vi "JTAG ADCScope.vi"() -> ()   [LabVIEW 2009]
panel:
  in  "stop 2":bool
  in  "Sample-Input Polarity":enum16{"Non-Inverted", "Inverted"}(ring)
  in  "Sample-Input Source Select":T1(ring)
  in  "ADC12 Clock Divider":T2(ring)
  in  "ADC12 Clock Source":enum16{"ADC12OSC", "ACLK", "MCLK", "SMCLK"}(ring)=enum."MCLK"
  in  "Update Delay (mS)":u32=100
  in  "Sample-Hold Trigger Source":enum16{"Sample-Input Signal", "Sampling Timer"}(ring)=enum."Sampling Timer"
  in  "MEM8-MEM15":T3(ring)
  in  "MEM0-MEM7":T3(ring)
  in  "Reference Generator":T4(ring)
  in  "Tab Control":enum32{"Single Channel", "Quad Channel"}(tab)
  out "ARG 7S":u16 format="%04x"
  out "Waveform Chart - Single Channel":u16(graph)
  in  "Select Voltage References (MEM0 Single)":T5(ring)
  in  "Input Channel Select (MEM0 Single)":T6(ring)
  in  "Select Voltage References (MEM3)":T5(ring)
  in  "Input Channel Select (MEM3)":T6(ring)
  in  "Select Voltage References (MEM2)":T5(ring)
  in  "Input Channel Select (MEM2)":T6(ring)
  in  "Select Voltage References (MEM1)":T5(ring)
  in  "Input Channel Select (MEM1)":T6(ring)
  out "Waveform Chart - 4 Channel":cluster{u16, u16, u16, u16}(graph)
  in  "Select Voltage References (MEM0)":T5(ring)
  in  "Input Channel Select (MEM0)":T6(ring)
  out "ARG 7M":u16 format="%04x"
  out "ARG 6M":u16 format="%04x"
  out "ARG 5M":u16 format="%04x"
  out "ARG 4M":u16 format="%04x"
  in  "stop":bool
  # "Sample and Hold Duration (ADC12 Clocks)"
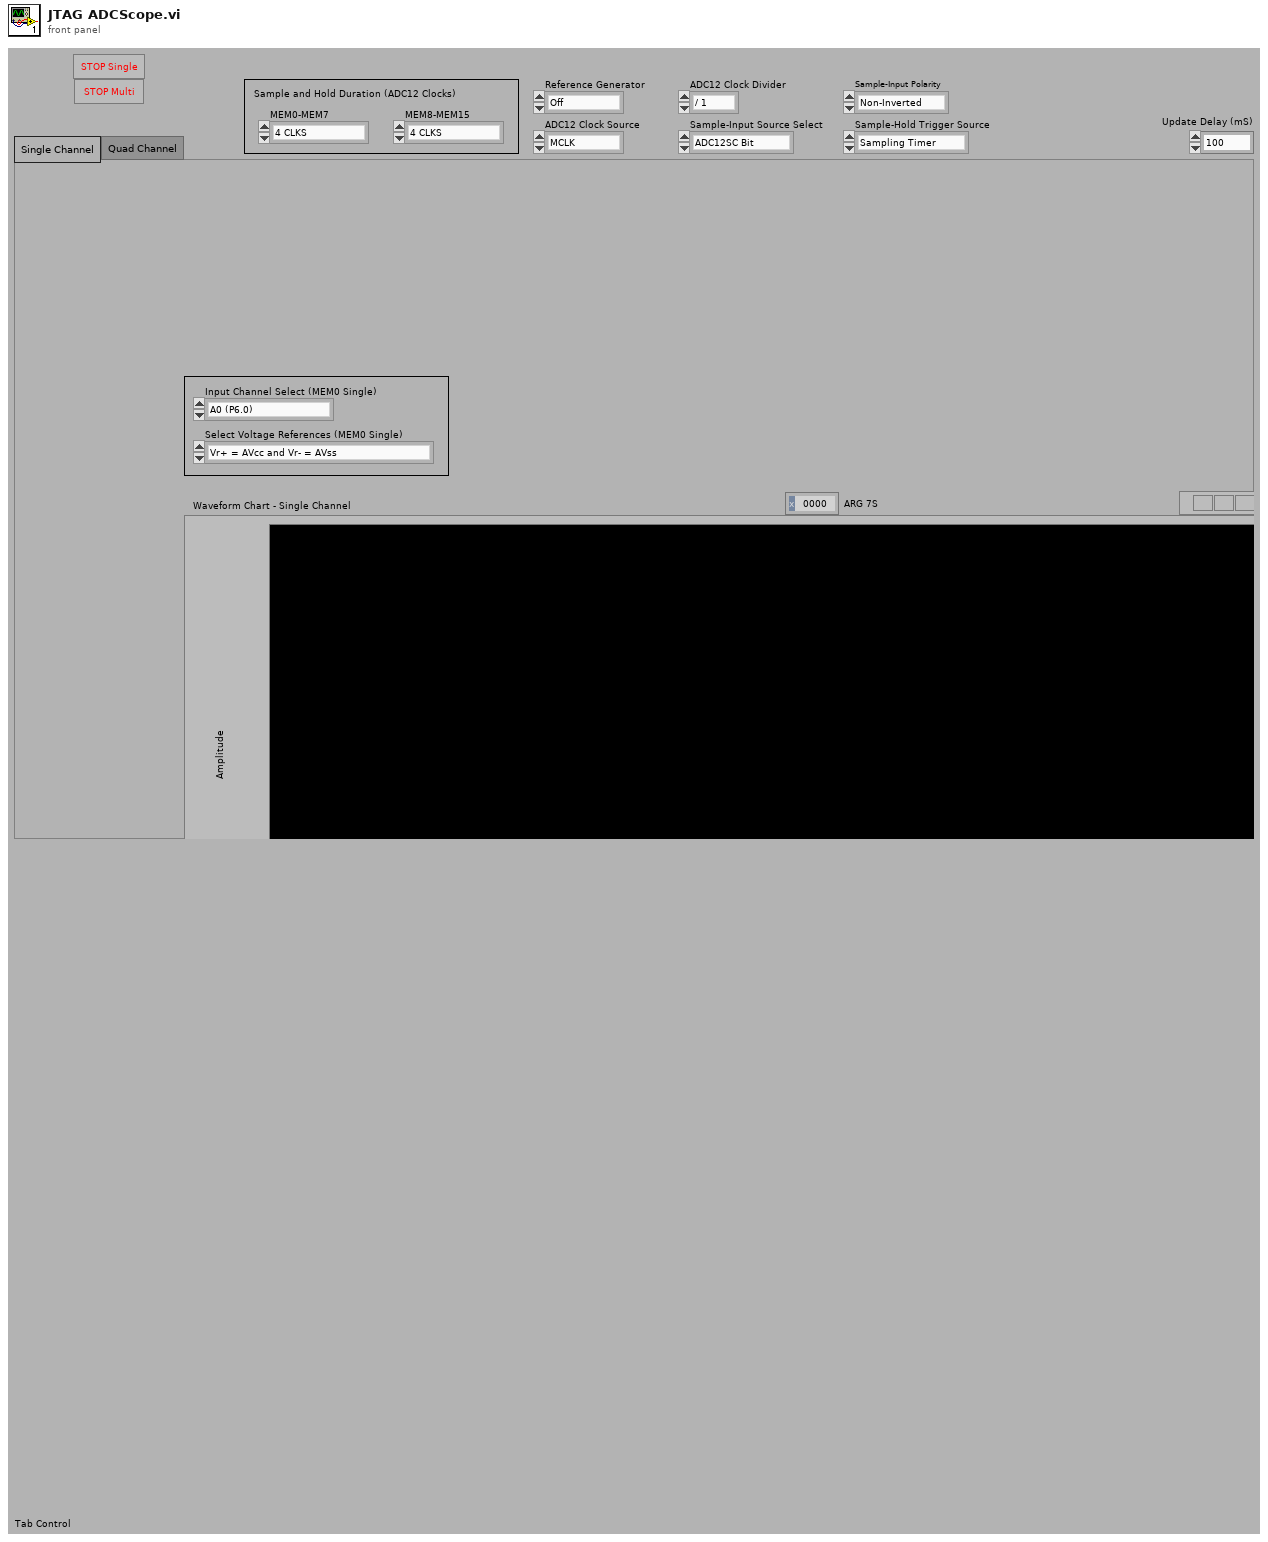
[diagram p1: front panel]
types:
  T1 = enum16{"ADC12SC Bit", "Timer_A OUT1", "Timer_B OUT0", "Timer_B OUT1"}
  T2 = enum16{"/ 1", "/ 2", "/ 3", "/ 4", "/ 5", "/ 6", "/ 7", "/ 8"}
  T3 = enum16{"4 CLKS", "8 CLKS", "16 CLKS", "32 CLKS", "64 CLKS", "96 CLKS", "128 CLKS", "192 CLKS", "256 CLKS", "384 CLKS", "512 CLKS", "768 CLKS", "1024 CLKS", "1024 CLKS (13)", "1024 CLKS (14)", "1024 CLKS (15)"}
  T4 = enum16{"Off", "ON - 1.5 V", "Off (2)", "ON - 2.5 V"}
  T5 = enum16{"Vr+ = AVcc and Vr- = AVss", "Vr+ = Vref+ and Vr-  = AVss", "Vr+ = Ve ref+ and Vr- = AVss", "Vr+ = Ve ref+ and Vr- = AVss (3)", "Vr+ = AVcc and Vr- = Vref- / Ve ref-", "Vr+ = Vref+ and Vr- = Vref- / Ve ref-", "Vr+ = Ve ref+ and Vr- = Vref- / Ve ref-", "Vr+ = Ve ref+ and Vr- = Vref- / Ve ref- (7)"}
  T6 = enum16{"A0 (P6.0)", "A1 (P6.1)", "A2 (P6.2)", "A3 (P6.3)", "A4 (P6.4)", "A5 (P6.5)", "A6 (P6.6)", "A7 (P6.7)", "Ve ref+", "V ref- / Ve ref-", "Temperature Diode", "(AVcc - AVss) / 2", "GND", "GND (13)", "GND (14)", "GND (15)"}
  T7 = enum8{"PORT_OUT", "PORT_SEL", "PORT_RES_EN", "READ_PORT", "PORT_DIR", "SET_LCM", "PLUTO_WRITE_SINGLE", "PLUTO_READ_SINGLE", "PLUTO_WRITE_MASK", "STIM_POWER_UP", "STIM_POWER_DN", "SATURN_WRITE_SINGLE", "SATURN_READ_SINGLE", "SATURN_WRITE_BLOCK", "SATURN_READ_BLOCK", "SATURN_WRITE_MASK", "MICS_POWER_UP", "MICS_POWER_DN", "MICS_WRITE_SINGLE", "MICS_READ_SINGLE", "MICS_WRITE_BLOCK", "MICS_READ_BLOCK", "MICS_WRITE_MASK", "MEM_POWER_UP", "MEM_POWER_DN", "MEM_WRITE_SINGLE", "MEM_READ_SINGLE", "MEM_WRITE_BLOCK", "MEM_READ_BLOCK", "MEM_WRITE_MASK", "MEM_WRITE_SR", "MEM_READ_SR", "MEM_OPCODE", "INIT_VARIABLES", "DCO -> 1 MHz", "DCO -> 8 MHz", "START_STIM_CLK", "STOP_STIM_CLK", "PULSE_STIM_CLK", "PULSE_STIM_SCK", "SINGLE_ADC12", "SINGLE_ADC12_REPEAT", "MULTI_ADC12", "MULTI_ADC12_REPEAT", "Disable_ADC12", "READ_IO_VARIABLES"}
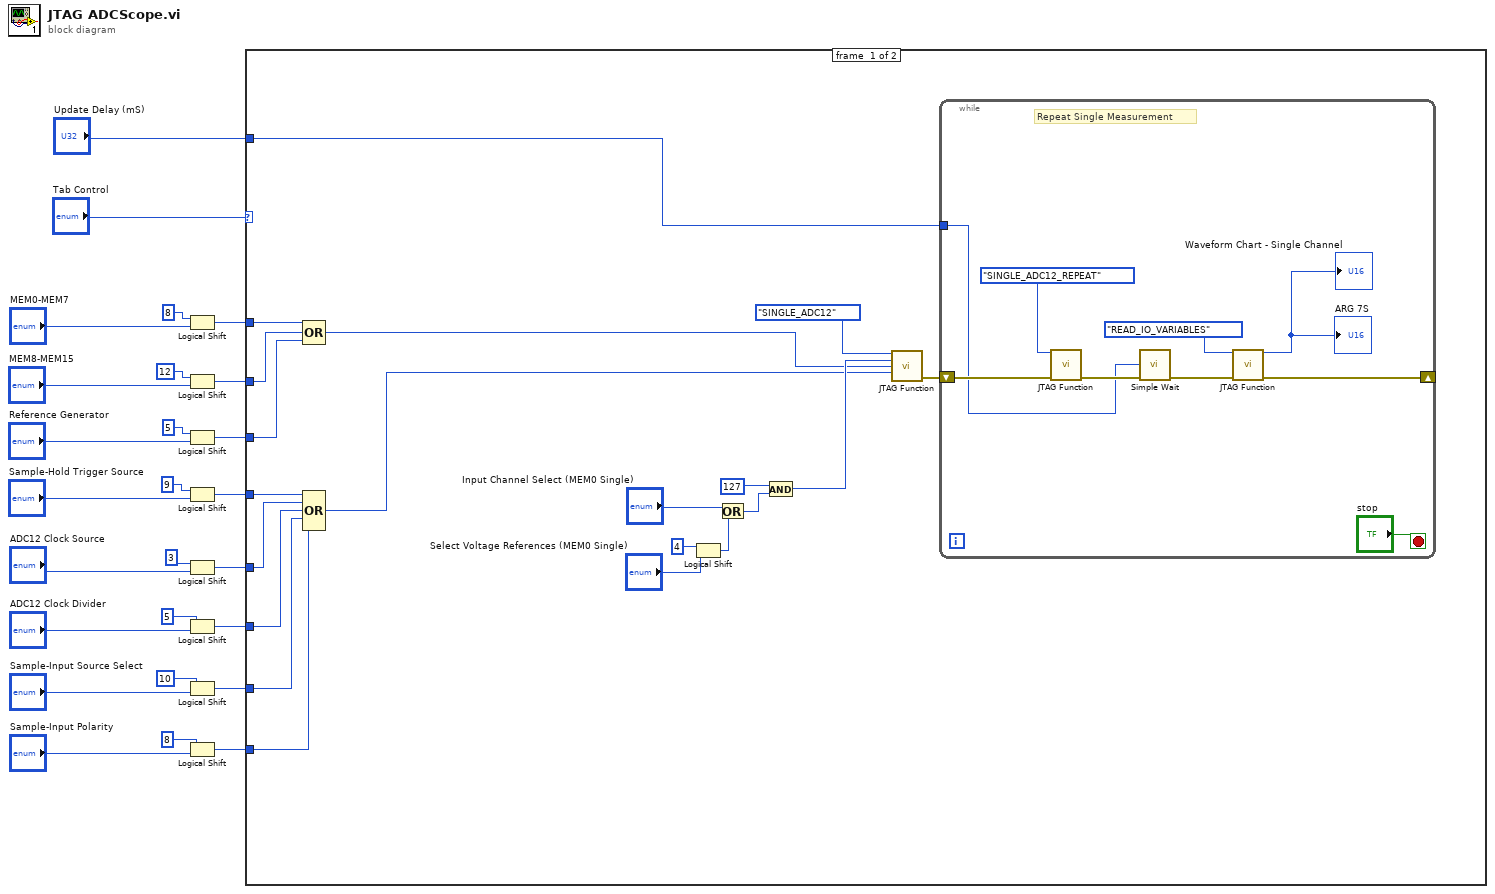
[diagram p0: block diagram]
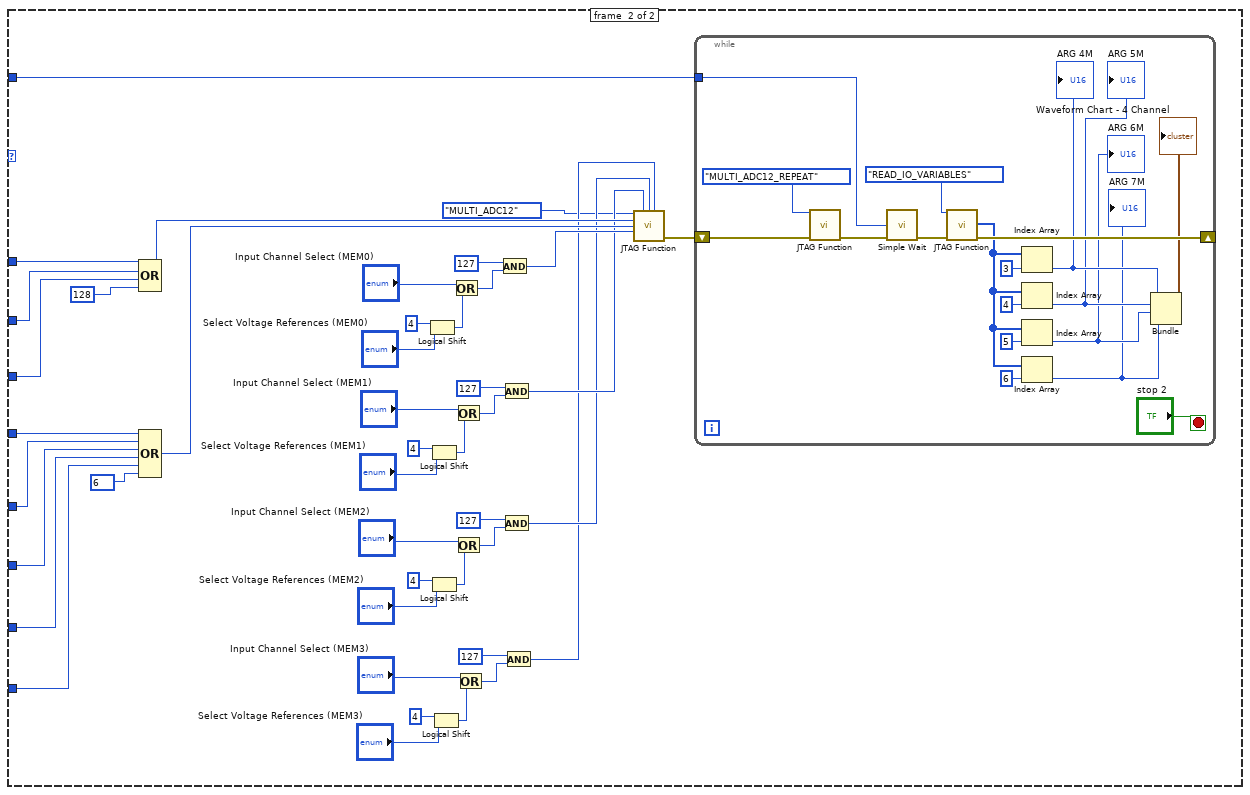
[diagram p2: hidden frame]
diagram:
  n1 = Logical Shift(y=i16 8, x="MEM0-MEM7") -> (x << y=w16:u32)
  n2 = Logical Shift(y=i16 12, x="MEM8-MEM15") -> (x << y=w15:u32)
  n3 = Logical Shift(y=i16 5, x="Reference Generator") -> (x << y=w14:u32)
  n4 = Logical Shift(y=i16 9, x="Sample-Hold Trigger Source") -> (x << y=w5:u32)
  n5 = Logical Shift(y=i16 3, x="ADC12 Clock Source") -> (x << y=w1:u32)
  n6 = Logical Shift(y=i16 5, x="ADC12 Clock Divider") -> (x << y=w2:u32)
  n7 = Logical Shift(y=i16 10, x="Sample-Input Source Select") -> (x << y=w3:u32)
  n8 = Logical Shift(y=i16 8, x="Sample-Input Polarity") -> (x << y=w4:u32)
  n9 = case shown="\"Single Channel\", Default" "Tab Control" {
    tunnel: "Update Delay (mS)" -> [w46 w98]
    tunnel: w16 -> [w39 w97]
    tunnel: w15 -> [w38 w96]
    tunnel: w14 -> [w37 w95]
    tunnel: w5 -> [w36 w94]
    tunnel: w4 -> [w35 w90]
    tunnel: w3 -> [w34 w91]
    tunnel: w2 -> [w33 w92]
    tunnel: w1 -> [w32 w93]
    frame #0 {
      n10 = Compound Arithmetic op=OR(w39, w38, w37) -> (w30:u32)
      n11 = Compound Arithmetic op=OR(w36, w32, w33, w34, w35) -> (w29:u32)
      n12 = Logical Shift(y=i16 4, x="Select Voltage References (MEM0 Single)") -> (x << y=w40:u32)
      n13 = Or(x="Input Channel Select (MEM0 Single)", y=w40) -> (x .or. y?=w44:u32)
      n14 = And(x=u8 127, y=w44) -> (x .and. y?=w31:u32)
      n15 = call "JTAG Function.vi"("Enum"=T7."SINGLE_ADC12", "ARG 1"=w31, "ARG 2"=w30, "ARG 3"=w29) -> ("error out"=w28:errorcluster)  [unwired: 9 in, 2 out]
      n16 = while {
        tunnel: w46 -> [w49]
        shift-right: [w54] -> _
        shift-left: w28 -> [w53]
        stop <- "stop" stop-if-true
        # "Repeat Single Measurement"
        n17 = call "JTAG Function.vi"("Enum"=T7."SINGLE_ADC12_REPEAT", "error in (no error)"=w53) -> ("error out"=w51:errorcluster)  [unwired: 11 in, 2 out]
        n18 = call "Simple Wait.vi"("mS"=w49, "error in"=w51) -> ("error out"=w50:errorcluster)  [unwired: 12 in, 1 out]
        n19 = call "JTAG Function.vi"("Enum"=T7."READ_IO_VARIABLES", "error in (no error)"=w50) -> ("ARG 7"=→"ARG 7S" →"Waveform Chart - Single Channel":u16, "error out"=w54:errorcluster)  [unwired: 11 in, 1 out]
      }
    }
    frame #1 {
      n20 = Compound Arithmetic op=OR(w97, w96, w95, u16 128) -> (w88:u32)
      n21 = Compound Arithmetic op=OR(w94, w93, w92, w91, w90, u16 6) -> (w87:u32)
      n22 = Logical Shift(y=i16 4, x="Select Voltage References (MEM0)") -> (x << y=w83:u32)
      n23 = Logical Shift(y=i16 4, x="Select Voltage References (MEM1)") -> (x << y=w79:u32)
      n24 = Logical Shift(y=i16 4, x="Select Voltage References (MEM2)") -> (x << y=w75:u32)
      n25 = Logical Shift(y=i16 4, x="Select Voltage References (MEM3)") -> (x << y=w71:u32)
      n26 = Or(x="Input Channel Select (MEM0)", y=w83) -> (x .or. y?=w85:u32)
      n27 = Or(x="Input Channel Select (MEM1)", y=w79) -> (x .or. y?=w81:u32)
      n28 = Or(x="Input Channel Select (MEM2)", y=w75) -> (x .or. y?=w77:u32)
      n29 = Or(x="Input Channel Select (MEM3)", y=w71) -> (x .or. y?=w73:u32)
      n30 = And(x=u8 127, y=w85) -> (x .and. y?=w62:u32)
      n31 = And(x=u8 127, y=w81) -> (x .and. y?=w61:u32)
      n32 = And(x=u8 127, y=w77) -> (x .and. y?=w60:u32)
      n33 = And(x=u8 127, y=w73) -> (x .and. y?=w59:u32)
      n34 = call "JTAG Function.vi"("Enum"=T7."MULTI_ADC12", "ARG 4"=w61, "ARG 5"=w60, "ARG 6"=w59, "ARG 1"=w88, "ARG 2"=w87, "ARG 3"=w62) -> ("error out"=w89:errorcluster)  [unwired: 6 in, 2 out]
      n35 = while {
        tunnel: w98 -> [w113]
        shift-right: [w111] -> _
        shift-left: w89 -> [w112]
        stop <- "stop 2" stop-if-true
        n36 = call "JTAG Function.vi"("Enum"=T7."MULTI_ADC12_REPEAT", "error in (no error)"=w112) -> ("error out"=w114:errorcluster)  [unwired: 11 in, 2 out]
        n37 = call "Simple Wait.vi"("mS"=w113, "error in"=w114) -> ("error out"=w115:errorcluster)  [unwired: 12 in, 1 out]
        n38 = call "JTAG Function.vi"("Enum"=T7."READ_IO_VARIABLES", "error in (no error)"=w115) -> ("ARG1-ARG7"=w109:u16[], "error out"=w111:errorcluster)  [unwired: 11 in, 1 out]
        n39 = Index Array(array=w109, index=3) -> (element=w104:u16)
        "ARG 4M" <- w104
        n40 = Index Array(array=w109, index=4) -> (element=w103:u16)
        "ARG 5M" <- w103
        n41 = Index Array(array=w109, index=5) -> (element=w102:u16)
        "ARG 6M" <- w102
        n42 = Index Array(array=w109, index=6) -> (element=w101:u16)
        "ARG 7M" <- w101
        n43 = Bundle(w104, w103, w102, w101) -> (→"Waveform Chart - 4 Channel":cluster{u16, u16, u16, u16})  [unwired: 1 in]
      }
    }
  }
